vi "Tree Create Item With Symbol and Color.vi"(5 "Color":u32, 7 "Symbol":i32=37, 8 "error in (no error)":errorcluster, 9 "Item Text":string, 10 "Parent Tag":string, 11 "TreeControl in":refnum<vi>) -> (0 "error out":errorcluster, 2 "Created Tag":string, 3 "TreeControl out":refnum<vi>)   [LabVIEW 2017]
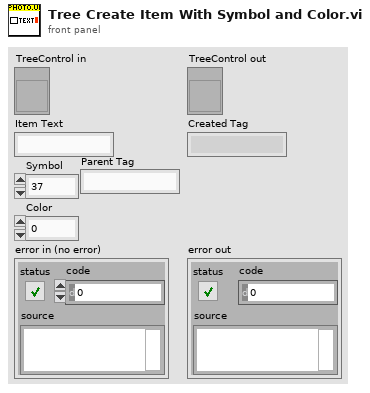
[diagram p1: front panel]
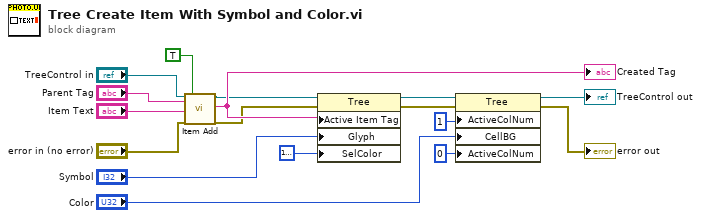
[diagram p0: block diagram]
diagram:
  n1 = call <instrlib>:"Item Add.vi"("Tree Reference In"="TreeControl in", "Parent Tag (Current)"="Parent Tag", "New Text Value"="Item Text", "error in (no error)"="error in (no error)", "Child Only?"=TRUE) -> ("Tree Reference Out"=w15:refnum<vi>, "Created Tag"=w17:string, "error out"=w16:errorcluster)  [unwired: 12 in]
  "Created Tag" <- w17
  n2 = property class="Tree"(reference=w15, error in=w16, "Active Item Tag"=w17, "Glyph"="Symbol", "SelColor"=u32 16777216) -> (reference out=w9:refnum<vi>, error out=w6:errorcluster)
  n3 = property class="Tree"(reference=w9, error in=w6, "ActiveColNum"=1 ("Active Cell:Active Column Number"), "CellBG"="Color", "ActiveColNum"=0 ("Active Cell:Active Column Number")) -> (reference out=→"TreeControl out":refnum<vi>, error out=→"error out":errorcluster)
